vi "Write Libraries.vi"(10 "Libraries":T1, 11 "Project in":refnum<class "Project.lvclass">) -> (3 "Project out":refnum<class "Project.lvclass">)   [LabVIEW 2016, in "Project.lvclass"]
uses:
  Project.lvclass
  Project.lvclass/Project.ctl
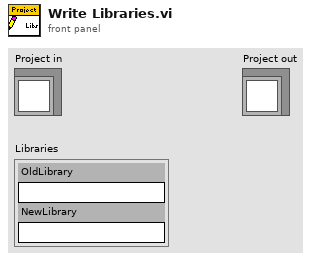
[diagram p1: front panel]
types:
  T1 = cluster{"OldLibrary":string, "NewLibrary":string}
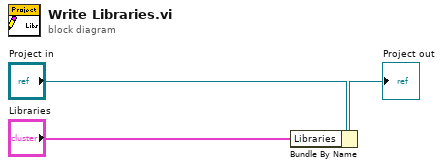
[diagram p0: block diagram]
diagram:
  n1 = Bundle By Name(cluster="Project in", "Libraries"="Libraries") -> (→"Project out":refnum<class "Project.lvclass">)
